vi "Read Process Step Configs.vi"(8 "error in (no error)":errorcluster, 11 "Process Settings in":refnum<class "Process Settings.lvclass">) -> (0 "error out":errorcluster, 2 "Process Step Configs":T1[](array[typedef]), 3 "Process Settings out":refnum<class "Process Settings.lvclass">)   [LabVIEW 2017, in "Process Settings.lvclass"]
uses:
  Process Settings.lvclass
  Type Defs/Process Step Description.ctl
  Type Defs/Item.ctl
  Type Defs/Units.ctl
  Process Settings.lvclass/Process Settings.ctl
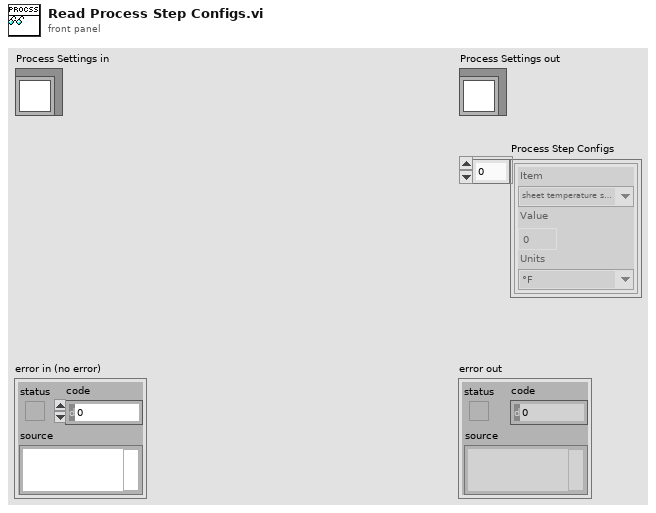
[diagram p1: front panel]
types:
  T1 = typedef "Process Settings.lvclass/Process Step Description.ctl" = cluster{"Item":T2, "Value":dbl, "Units":T3}
  T2 = typedef "Process Settings.lvclass/Item.ctl" = enum16{"", "sheet temperature setpoint", "sheet heating time", "temp element setpoint", "chamber pressure", "saturation time"}
  T3 = typedef "Process Settings.lvclass/Units.ctl" = enum16{"°F", "°C", "Seconds", "Minutes", "PSIA"}
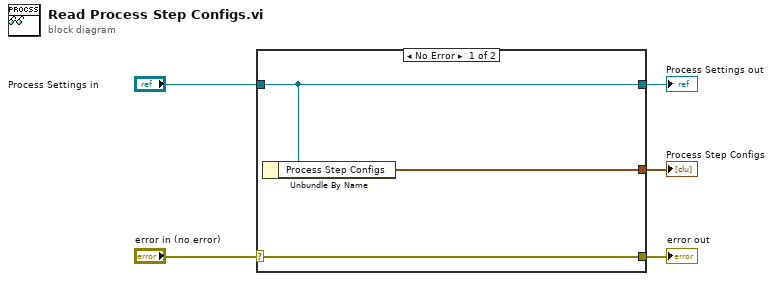
[diagram p0: block diagram]
diagram:
  n1 = case shown="No Error" "error in (no error)" {
    selector: "error in (no error)" -> [w8 w9]
    tunnel: [w8 w9] -> w4
    tunnel: [w7 w10] -> w2
    tunnel: "Process Settings in" -> [w7 w10]
    tunnel: [w6 _] -> w1
    frame No Error {
      n2 = Unbundle By Name(w7) -> ("Process Step Configs"=w6:T1[])
    }
    frame Error {
    }
  }
  "error out" <- w4
  "Process Settings out" <- w2
  "Process Step Configs" <- w1
